vi "CRC16-发送校验.vi"(1 "净数据":string) -> (0 "完整输出":string)   [LabVIEW 2017]
panel:
  out "CRC16":string
  out "CRCL":string
  out "CRCH":string
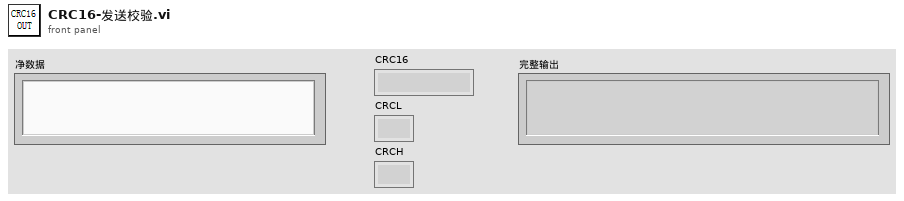
[diagram p1: front panel]
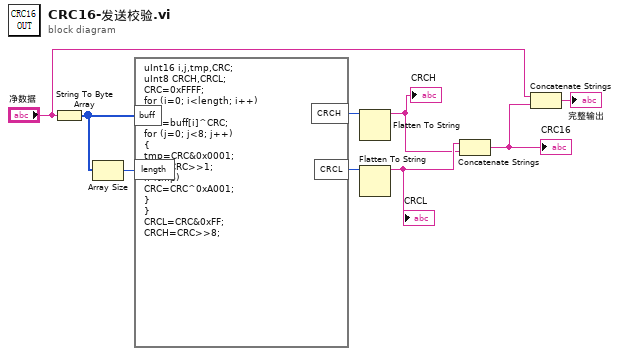
[diagram p0: block diagram]
diagram:
  n1 = String To Byte Array(string="净数据") -> (unsigned byte array=w9:u8[])
  n2 = Array Size(array=w9) -> (size(s)=w8:i32)
  n3 = formula code="uInt16 i,j,tmp,CRC;\nuInt8 CRCH,CRCL;\nCRC=0xFFFF;\nfor (i=0; i<length; i++)\n{\nCRC=buff[i]^CRC;\nfor (j=0; j<8; j++)\n{\ntmp=CRC&0x0001;\nCRC=CRC>>1;\nif (tmp) \nCRC=CRC^0xA001;\n}\n}\nCRCL=CRC&0xFF;\nCRCH=CRC>>8;"("buff"=w9, "length"=w8) -> ("CRCH"=w7:u8, "CRCL"=w6:u8)
  n4 = Flatten To String(anything=w7) -> (data string=w4:string)  [unwired: 3 in, 2 out]
  "CRCH" <- w4
  n5 = Flatten To String(anything=w6) -> (data string=w5:string)  [unwired: 3 in, 2 out]
  "CRCL" <- w5
  n6 = Concatenate Strings(w5, w4) -> (w3:string)
  "CRC16" <- w3
  n7 = Concatenate Strings("净数据", w3) -> (→"完整输出":string)
